vi "REalsense Cam Stream Start.vi"(7 "Use new Resolution? (F)":bool, 8 "error in (no error)":errorcluster, 9 "Resolution":u16(ring)=27 items=["424 x 240 @6fps", "424 x 240 @15fps", "424 x 240 @30fps", "424 x 240 @60fps", "424 x 240 @90fps", "480 x 270 @6fps", "480 x 270 @15fps", "480 x 270 @30fps", "480 x 270 @60fps", "480 x 270 @90fps", "640 x 360 @6fps", "640 x 360 @15fps", "640 x 360 @30fps", "640 x 360 @60fps", "640 x 360 @90fps", "640 x 480 @6fps", "640 x 480 @15fps", "640 x 480 @30fps", "640 x 480 @60fps", "640 x 480 @90fps", "848 x 100 @100fps", "848 x 480 @6fps", "848 x 480 @15fps", "848 x 480 @30fps", "848 x 480 @60fps", "848 x 480 @90fps", "1280 x 720 @6fps", "1280 x 720 @15fps", "1280 x 720 @30fps", "1280 x 800 @15fps", "1280 x 800 @30fps"], 10 "Stream Type":T1=enum."Left IR", 11 "Realsense Cam in":refnum<class "Realsense Cam.lvclass">) -> (0 "error out":errorcluster, 3 "Realsense Cam out":refnum<class "Realsense Cam.lvclass">)   [LabVIEW 2018, in "Realsense Cam.lvclass"]
uses:
  Realsense Cam.lvclass
  Private/Stream Types Enum STYP.ctl
  Realsense Cam.lvclass/Realsense Cam.ctl
  Private/Activated Stream STYP.ctl
  Private/Stream STYP.ctl
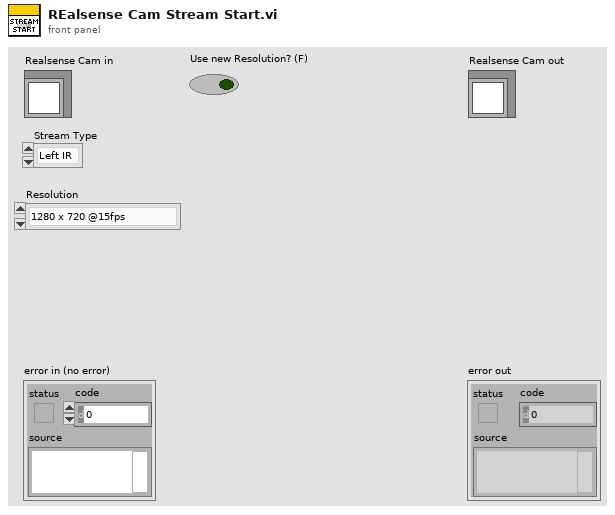
[diagram p1: front panel]
types:
  T1 = typedef "Realsense Cam.lvclass/Stream Types Enum STYP.ctl" = enum16{"Depth", "Left IR", "Right IR", "Color", "RGB Ext.", "Left IR Unrectified", "Right IR Unrectified"}
  T2 = typedef "Realsense Cam.lvclass/Activated Stream STYP.ctl" = cluster{"Stream Type":T1, "Resolution":u16, "Profile Handle":u64, "Stream":T3}
  T3 = typedef "Realsense Cam.lvclass/Stream STYP.ctl" = cluster{"Strings":string[], "Intrinsics":cluster{"width":i32, "height":i32, "fps":i32, "Profile":u64, "ppx":sgl, "ppy":sgl, "fx":sgl, "fy":sgl, "model":u32}[], "Current Data":cluster{"Depths":sgl[][], "Bytes":u8[], "Height":i32, "Width":i32}}
  T4 = cluster{"width":i32, "height":i32, "fps":i32, "Profile":u64, "ppx":sgl, "ppy":sgl, "fx":sgl, "fy":sgl, "model":u32}[]
  T5 = cluster{"width":i32, "height":i32, "fps":i32, "Profile":u64, "ppx":sgl, "ppy":sgl, "fx":sgl, "fy":sgl, "model":u32}
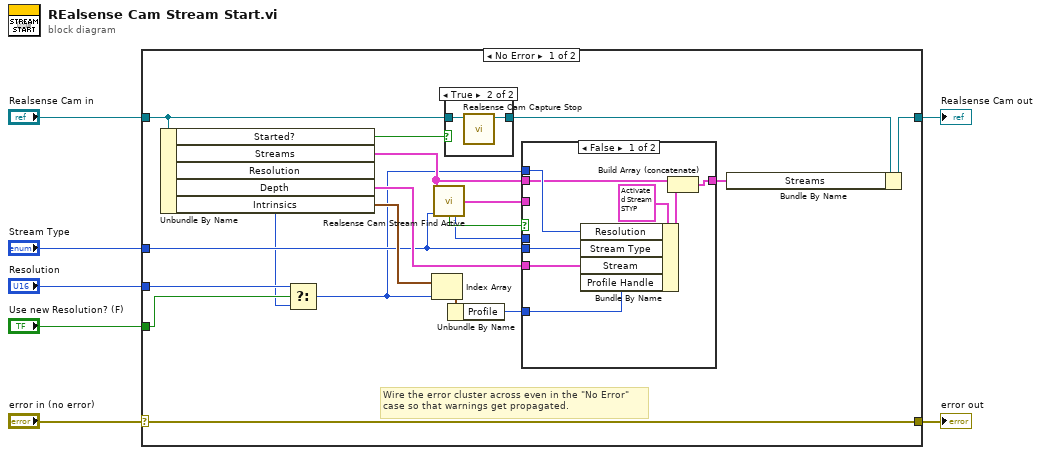
[diagram p0: block diagram]
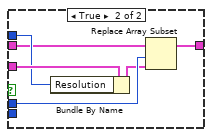
[diagram p2: hidden frame]
diagram:
  n1 = case shown="No Error" "error in (no error)" {
    selector: "error in (no error)" -> [w26 w45]
    tunnel: [w26 w45] -> w6
    tunnel: [w13 w44] -> w4
    tunnel: "Realsense Cam in" -> [w25 w44]
    tunnel: "Stream Type" -> [w12 _]
    tunnel: "Use new Resolution? (F)" -> [w11 _]
    tunnel: "Resolution" -> [w10 _]
    frame No Error {
      # "Wire the error cluster across even in the \"No Error\"\ncase so that warnings get propagated."
      n2 = Unbundle By Name(w25) -> ("Started?"=w24:bool, "Streams"=w20:T2[], "Resolution"=w9:u16, "Depth"=w19:T3, "Intrinsics"=w18:T4)
      n3 = Select(t=w10, s=w11, f=w9) -> (s? t:f=w8:u16)
      n4 = Index Array(array=w18, index=w8) -> (element=w17:T5)
      n5 = call "Realsense Cam Stream Find Active.vi"("Streams"=w20, "Stream Types"=w12) -> ("Activated Stream"=w21:T2, "Found?"=w23:bool, "Index"=w22:i32)  [unwired: 11 in]
      n6 = case shown="True" w24 {
        tunnel: w25 -> [w41 w43]
        tunnel: [w41 w42] -> w15
        frame False {
        }
        frame True {
          n7 = call-dynamic "Realsense Cam Capture Stop.vi"("Realsense Cam in"=w43) -> ("Realsense Cam out"=w42:refnum<class "Realsense Cam.lvclass">)  [unwired: 8 in, 2 out]
        }
      }
      n8 = Unbundle By Name(w17) -> ("Profile"=w16:u64)
      n9 = case shown="False" w23 {
        tunnel: w22 -> [_ w37]
        tunnel: w21 -> [_ w40]
        tunnel: w8 -> [w30 w39]
        tunnel: w20 -> [w29 w38]
        tunnel: w12 -> [w31 _]
        tunnel: [w27 w35] -> w14
        tunnel: w19 -> [w32 _]
        tunnel: w16 -> [w33 _]
        frame False {
          n10 = Bundle By Name(cluster=T2 {"Stream Type"=enum."Color", "Resolution"=17, "Profile Handle"=0, "Stream"={"Strings"=["424 x 240 @6fps", "424 x 240 @15fps", "424 x 240 @30fps", "424 x 240 @60fps", "424 x 240 @90fps", "480 x 270 @6fps", "480 x 270 @15fps", "480 x 270 @30fps", "480 x 270 @60fps", "480 x 270 @90fps", "640 x 360 @6fps", "640 x 360 @15fps", "640 x 360 @30fps", "640 x 360 @60fps", "640 x 360 @90fps", "640 x 480 @6fps", "640 x 480 @15fps", "640 x 480 @30fps", "640 x 480 @60fps", "640 x 480 @90fps", "848 x 480 @6fps", "848 x 480 @15fps", "848 x 480 @30fps", "848 x 480 @60fps", "848 x 480 @90fps", "1280 x 720 @6fps", "1280 x 720 @15fps", "1280 x 720 @30fps", "1920 x 1080 @15fps", "1920 x 1080 @25fps"], "Intrinsics"=[{"width"=424, "height"=240, "fps"=6, "Profile"=521311384, "ppx"=210.19093, "ppy"=123.56658, "fx"=317.53546, "fy"=317.53546, "model"=4}, {"width"=424, "height"=240, "fps"=15, "Profile"=521310104, "ppx"=210.19093, "ppy"=123.56658, "fx"=317.53546, "fy"=317.53546, "model"=4}, {"width"=424, "height"=240, "fps"=30, "Profile"=521314712, "ppx"=210.19093, "ppy"=123.56658, "fx"=317.53546, "fy"=317.53546, "model"=4}, {"width"=424, "height"=240, "fps"=60, "Profile"=521313688, "ppx"=210.19093, "ppy"=123.56658, "fx"=317.53546, "fy"=317.53546, "model"=4}, {"width"=424, "height"=240, "fps"=90, "Profile"=521315736, "ppx"=210.19093, "ppy"=123.56658, "fx"=317.53546, "fy"=317.53546, "model"=4}, {"width"=480, "height"=270, "fps"=6, "Profile"=521314968, "ppx"=237.96481, "ppy"=139.0124, "fx"=357.2274, "fy"=357.2274, "model"=4}, {"width"=480, "height"=270, "fps"=15, "Profile"=521318808, "ppx"=237.96481, "ppy"=139.0124, "fx"=357.2274, "fy"=357.2274, "model"=4}, {"width"=480, "height"=270, "fps"=30, "Profile"=521316504, "ppx"=237.96481, "ppy"=139.0124, "fx"=357.2274, "fy"=357.2274, "model"=4}, {"width"=480, "height"=270, "fps"=60, "Profile"=521322904, "ppx"=237.96481, "ppy"=139.0124, "fx"=357.2274, "fy"=357.2274, "model"=4}, {"width"=480, "height"=270, "fps"=90, "Profile"=521312152, "ppx"=237.96481, "ppy"=139.0124, "fx"=357.2274, "fy"=357.2274, "model"=4}, {"width"=640, "height"=360, "fps"=6, "Profile"=521314200, "ppx"=317.2864, "ppy"=185.34987, "fx"=476.3032, "fy"=476.3032, "model"=4}, {"width"=640, "height"=360, "fps"=15, "Profile"=521319320, "ppx"=317.2864, "ppy"=185.34987, "fx"=476.3032, "fy"=476.3032, "model"=4}, {"width"=640, "height"=360, "fps"=30, "Profile"=521319064, "ppx"=317.2864, "ppy"=185.34987, "fx"=476.3032, "fy"=476.3032, "model"=4}, {"width"=640, "height"=360, "fps"=60, "Profile"=521321112, "ppx"=317.2864, "ppy"=185.34987, "fx"=476.3032, "fy"=476.3032, "model"=4}, {"width"=640, "height"=360, "fps"=90, "Profile"=521318296, "ppx"=317.2864, "ppy"=185.34987, "fx"=476.3032, "fy"=476.3032, "model"=4}, {"width"=640, "height"=480, "fps"=6, "Profile"=521313176, "ppx"=316.38187, "ppy"=247.13316, "fx"=635.0709, "fy"=635.0709, "model"=4}, {"width"=640, "height"=480, "fps"=15, "Profile"=521321368, "ppx"=316.38187, "ppy"=247.13316, "fx"=635.0709, "fy"=635.0709, "model"=4}, {"width"=640, "height"=480, "fps"=30, "Profile"=521309592, "ppx"=316.38187, "ppy"=247.13316, "fx"=635.0709, "fy"=635.0709, "model"=4}, {"width"=640, "height"=480, "fps"=60, "Profile"=521320088, "ppx"=316.38187, "ppy"=247.13316, "fx"=635.0709, "fy"=635.0709, "model"=4}, {"width"=640, "height"=480, "fps"=90, "Profile"=521322648, "ppx"=316.38187, "ppy"=247.13316, "fx"=635.0709, "fy"=635.0709, "model"=4}, {"width"=848, "height"=480, "fps"=6, "Profile"=521315992, "ppx"=420.38187, "ppy"=247.13316, "fx"=635.0709, "fy"=635.0709, "model"=4}, {"width"=848, "height"=480, "fps"=15, "Profile"=521317272, "ppx"=420.38187, "ppy"=247.13316, "fx"=635.0709, "fy"=635.0709, "model"=4}, {"width"=848, "height"=480, "fps"=30, "Profile"=521310616, "ppx"=420.38187, "ppy"=247.13316, "fx"=635.0709, "fy"=635.0709, "model"=4}, {"width"=848, "height"=480, "fps"=60, "Profile"=521310360, "ppx"=420.38187, "ppy"=247.13316, "fx"=635.0709, "fy"=635.0709, "model"=4}, {"width"=848, "height"=480, "fps"=90, "Profile"=521306776, "ppx"=420.38187, "ppy"=247.13316, "fx"=635.0709, "fy"=635.0709, "model"=4}, {"width"=1280, "height"=720, "fps"=6, "Profile"=521320600, "ppx"=634.5728, "ppy"=370.69974, "fx"=952.6064, "fy"=952.6064, "model"=4}, {"width"=1280, "height"=720, "fps"=15, "Profile"=521310872, "ppx"=634.5728, "ppy"=370.69974, "fx"=952.6064, "fy"=952.6064, "model"=4}, {"width"=1280, "height"=720, "fps"=30, "Profile"=521320344, "ppx"=634.5728, "ppy"=370.69974, "fx"=952.6064, "fy"=952.6064, "model"=4}, {"width"=1920, "height"=1080, "fps"=15, "Profile"=521627576, "ppx"=951.85925, "ppy"=556.0496, "fx"=1428.9095, "fy"=1428.9095, "model"=4}, {"width"=1920, "height"=1080, "fps"=25, "Profile"=521617080, "ppx"=951.85925, "ppy"=556.0496, "fx"=1428.9095, "fy"=1428.9095, "model"=4}], "Current Data"={"Depths"=[], "Bytes"=[], "Height"=0, "Width"=0}}} ("Activated Stream"), "Resolution"=w30, "Stream Type"=w31, "Stream"=w32, "Profile Handle"=w33) -> (w28:T2)
          n11 = Build Array (concatenate)(w29, w28) -> (w27:T2[])
        }
        frame True {
          n12 = Bundle By Name(cluster=w40, "Resolution"=w39) -> (w36:T2)
          n13 = Replace Array Subset(array=w38, new element=w36, index=w37) -> (w35:T2[])
        }
      }
      n14 = Bundle By Name(cluster=w15, "Streams"=w14) -> (w13:refnum<class "Realsense Cam.lvclass">)
    }
    frame Error {
    }
  }
  "error out" <- w6
  "Realsense Cam out" <- w4
